vi "打码软件.vi"() -> ()   [LabVIEW 2014]
uses:
  <vilib>/Instr/_visa.llb/VISA Configure Serial Port (Instr).vi
  <vilib>/ptbypt/NI_PtbyPt.lvlib
panel:
  in  "监控":bool
  out "选项卡控件":enum32{"主选项卡", "监控"}(tab)
  in  "输入打标码后五位\n如：S0001":string
  in  "确定":bool
  out "当前打标码":string
  in  "手动打标":bool
  in  "停止":bool
  in  "退出":bool
  in  "PLC状态":bool
  out "串口通讯":bool
  out "PLC通讯":bool
  in  "返回":bool
  out "初始化回复":string
  out "打标模式回复":string
  out "初始条码":string
  out "打标V1写入回复":string
  out "打标V3写入回复":string
  out "开始打标写入回复":string
  out "停止打标回复":string
  in  "自动打标":bool
  out "错误输出 2":errorcluster caption="错误输出"
  out "元素":u32
  out "初始化文件回复":string
  # "SIC 打 标 软 件"
  # "自定义条码"
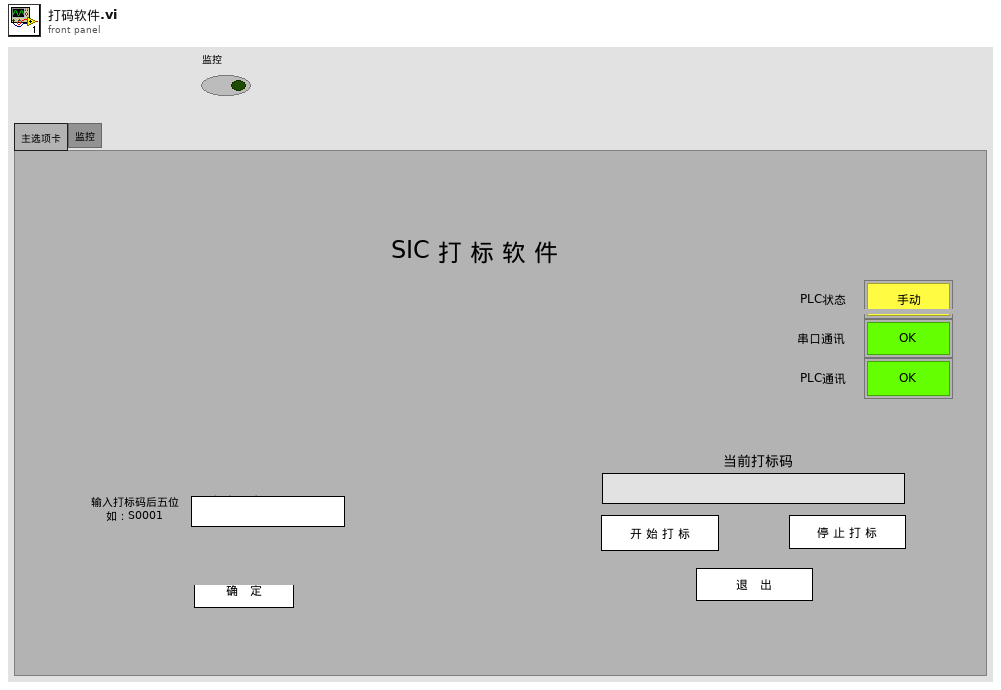
[diagram p1: front panel]
types:
  T1 = typedef "控件 1.ctl" = enum16{"通讯连接", "读PLC指令", "串口连接", "初始化", "打标模式", "事件", "错误", "退出"}
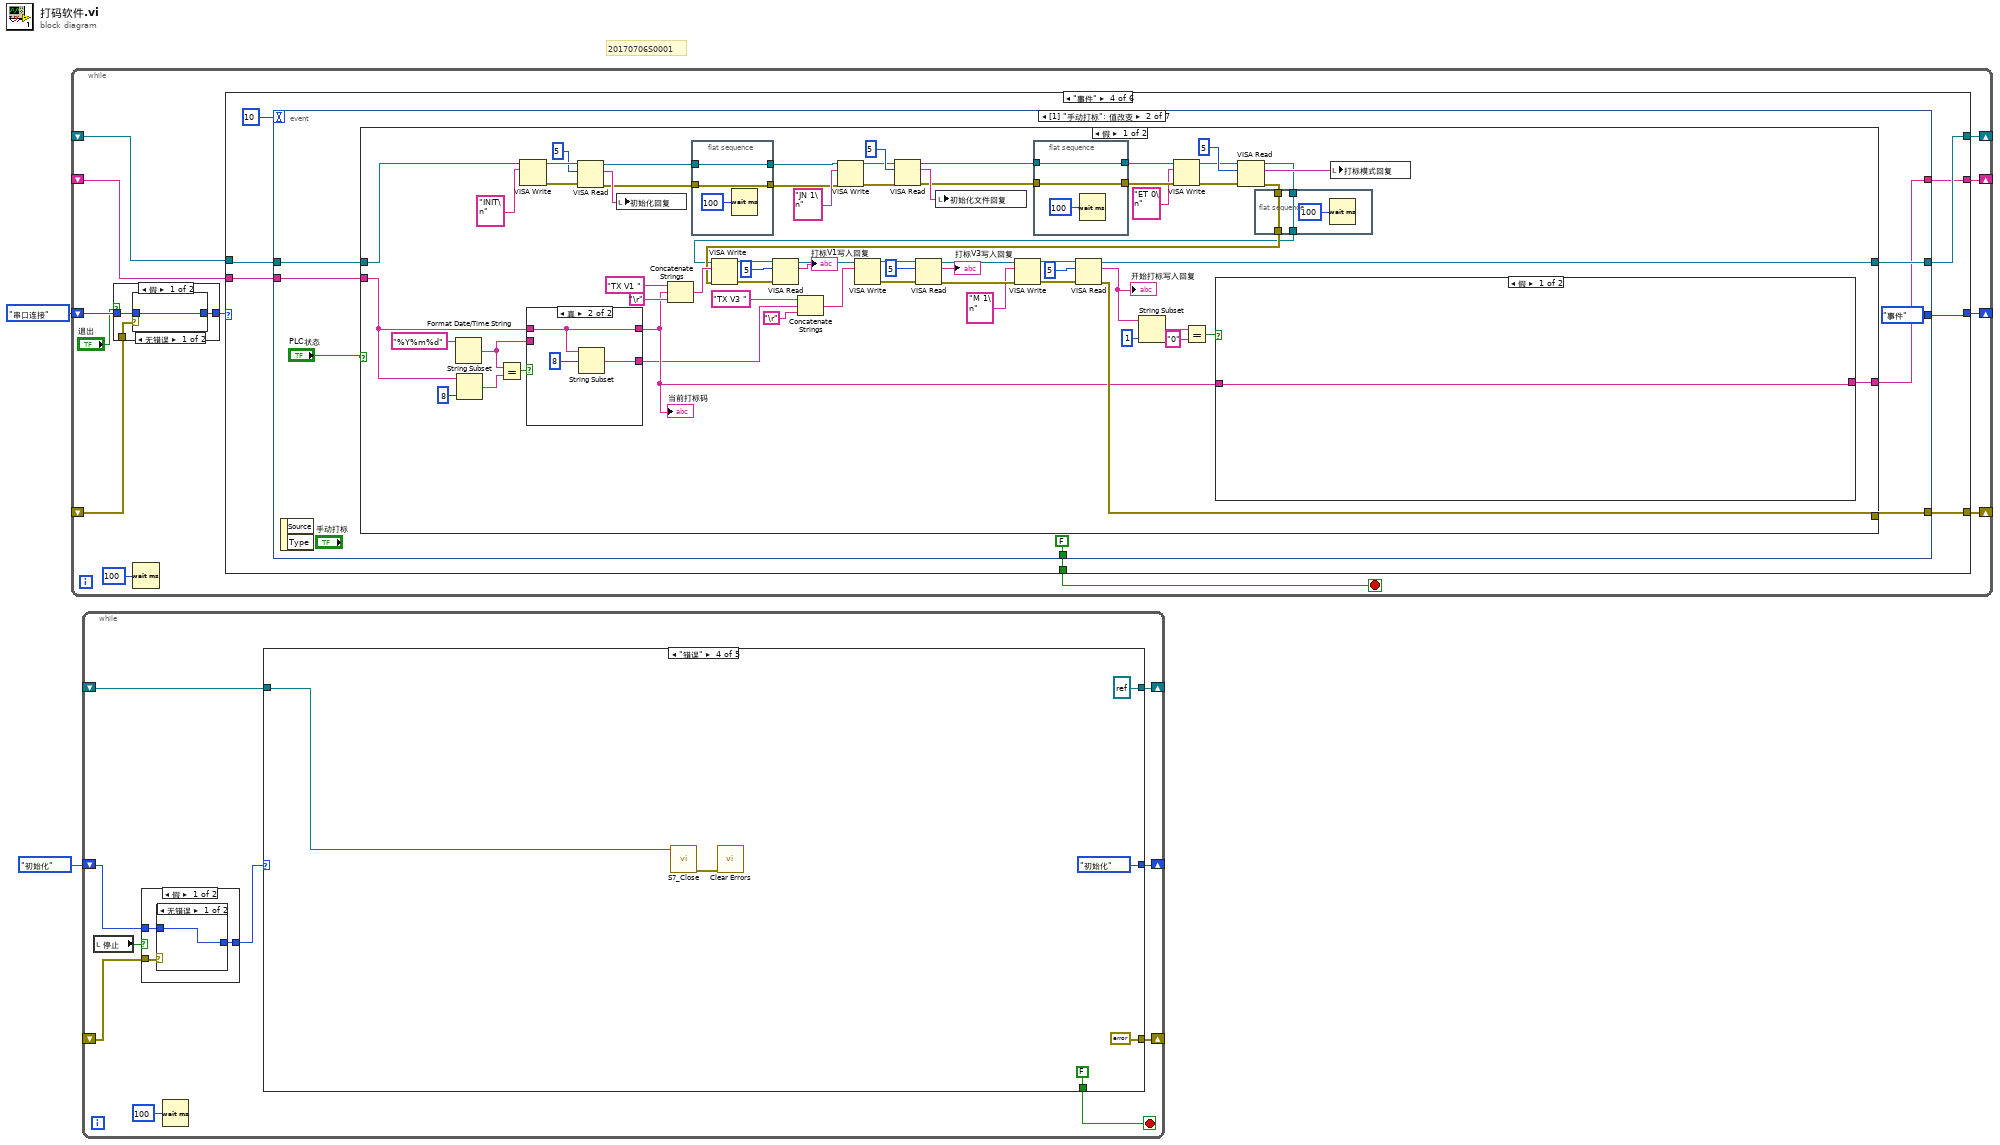
[diagram p0: block diagram]
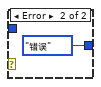
[diagram p2: hidden frame]
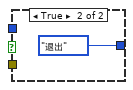
[diagram p3: hidden frame]
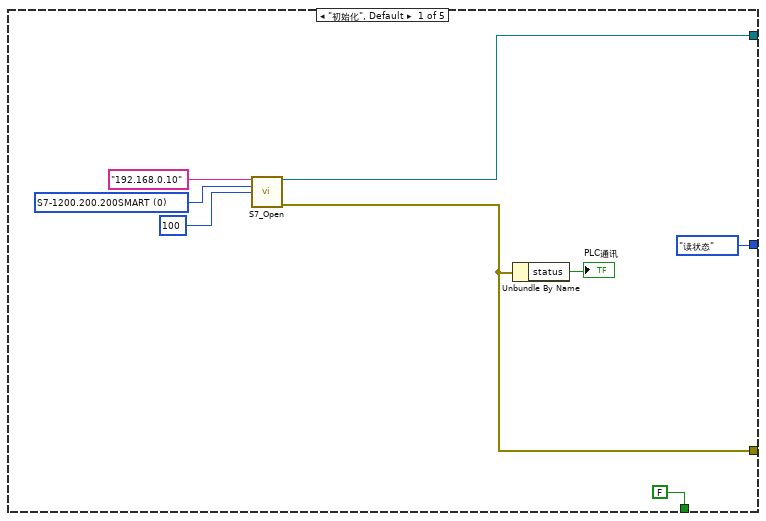
[diagram p4: hidden frame]
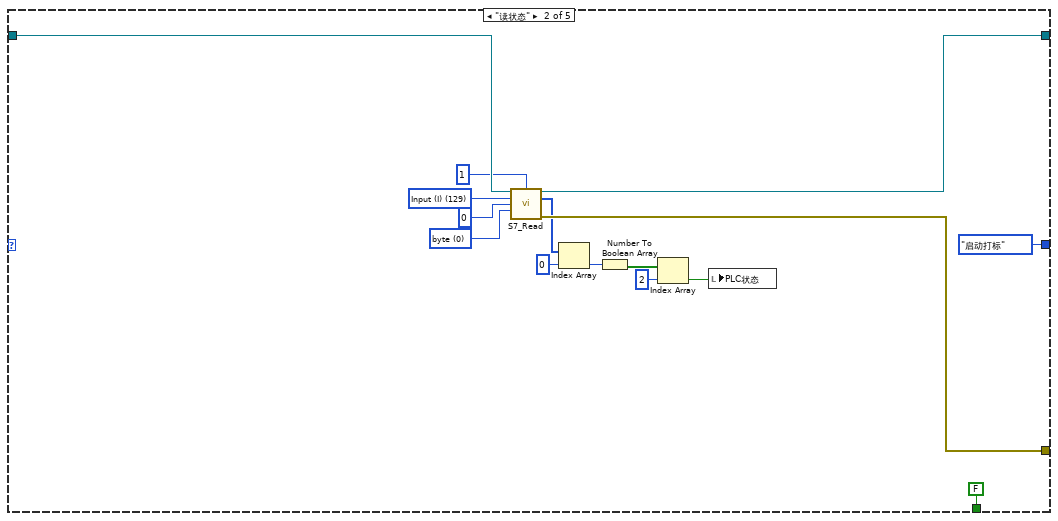
[diagram p5: hidden frame]
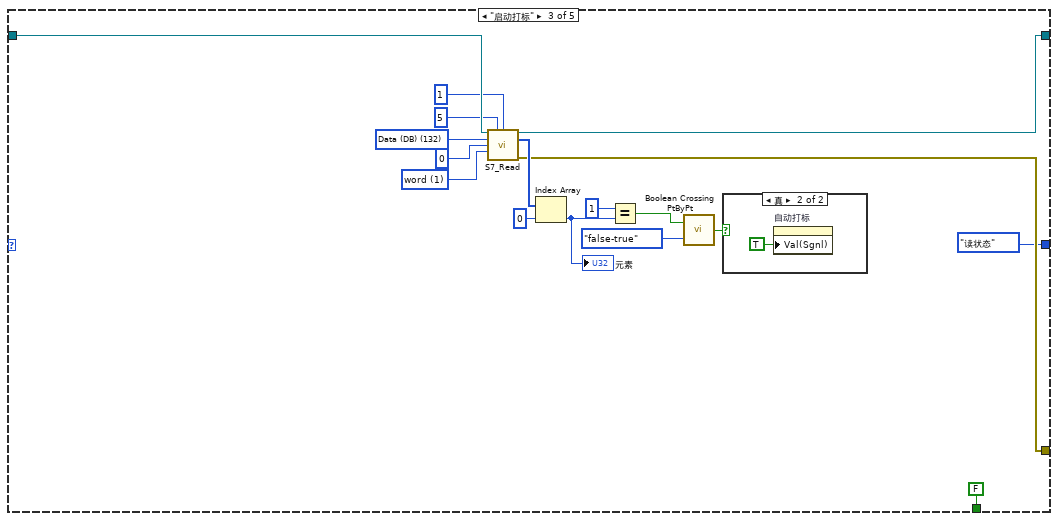
[diagram p6: hidden frame]
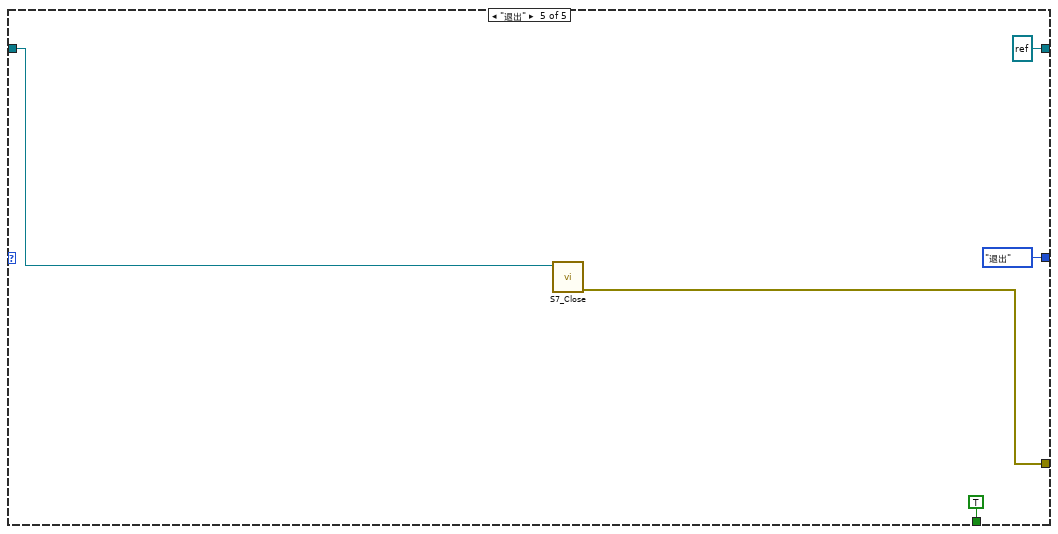
[diagram p8: hidden frame]
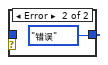
[diagram p9: hidden frame]
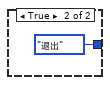
[diagram p10: hidden frame]
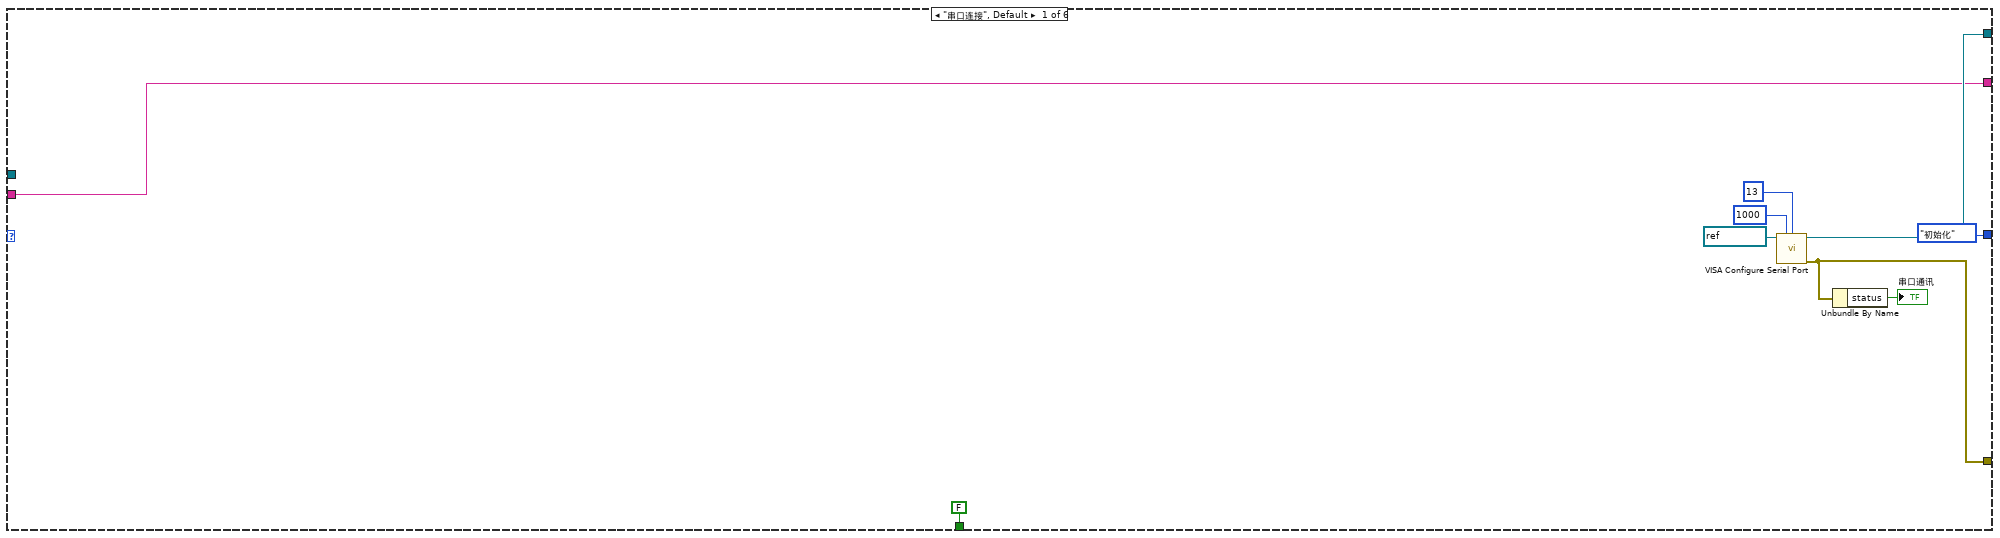
[diagram p11: hidden frame]
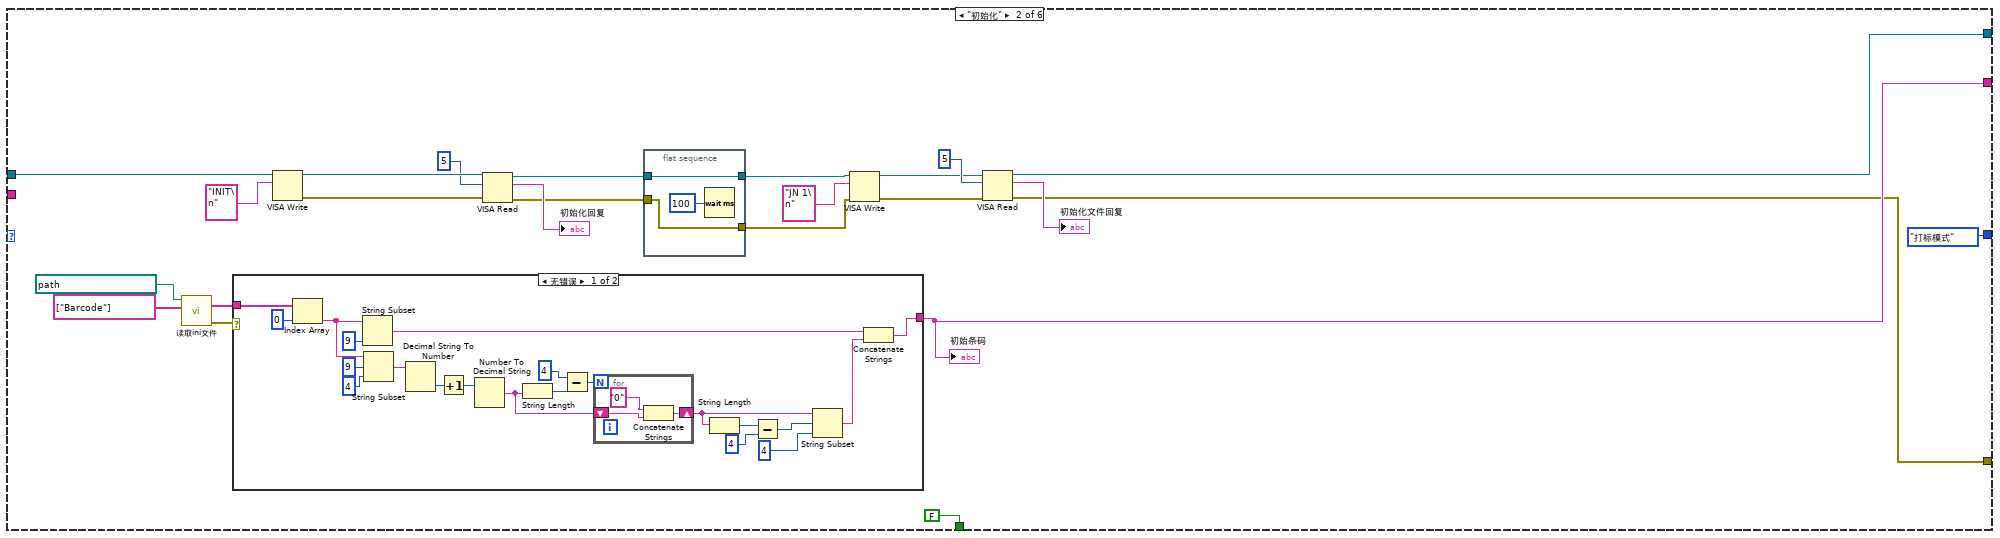
[diagram p12: hidden frame]
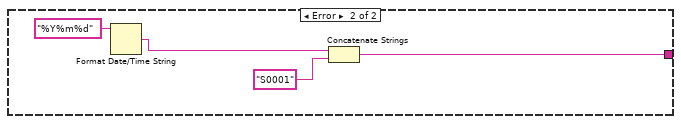
[diagram p13: hidden frame]
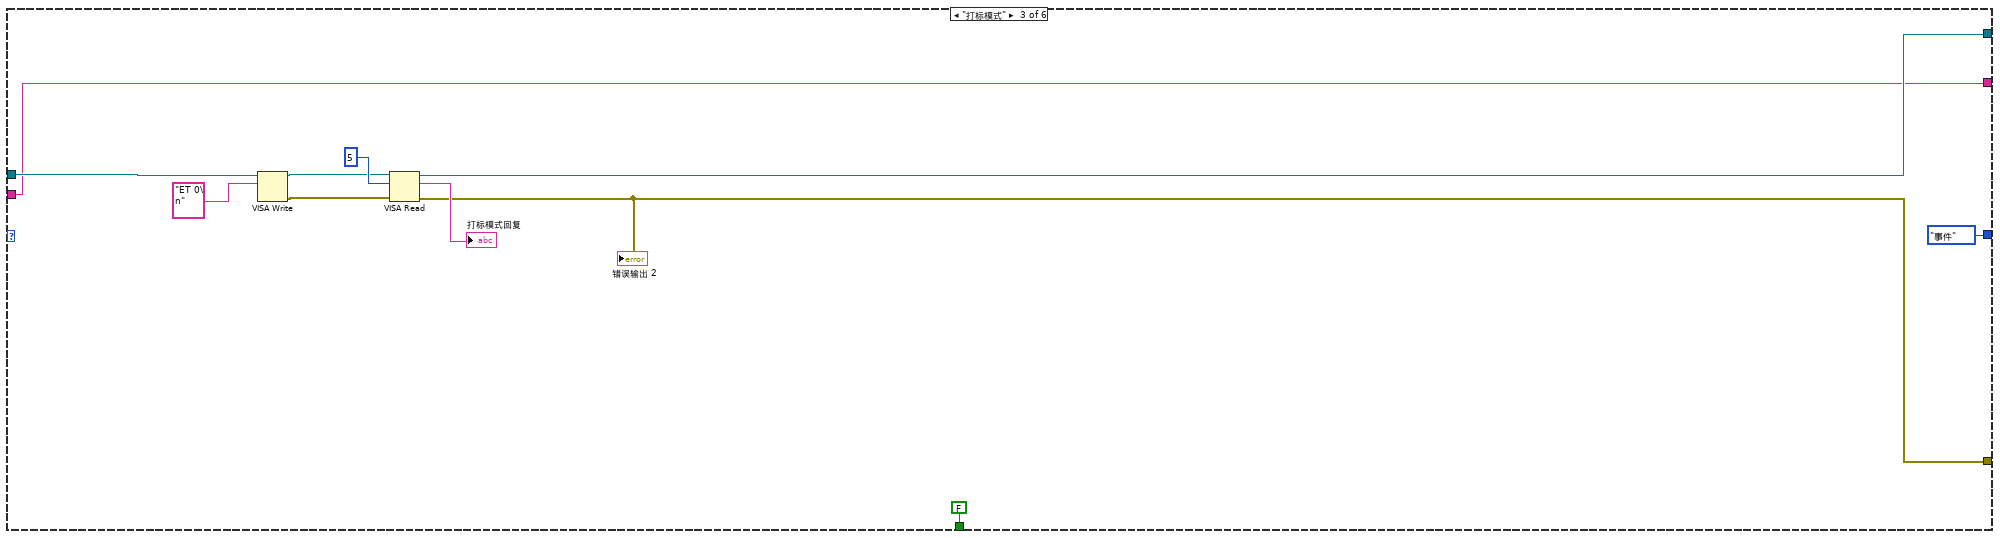
[diagram p14: hidden frame]
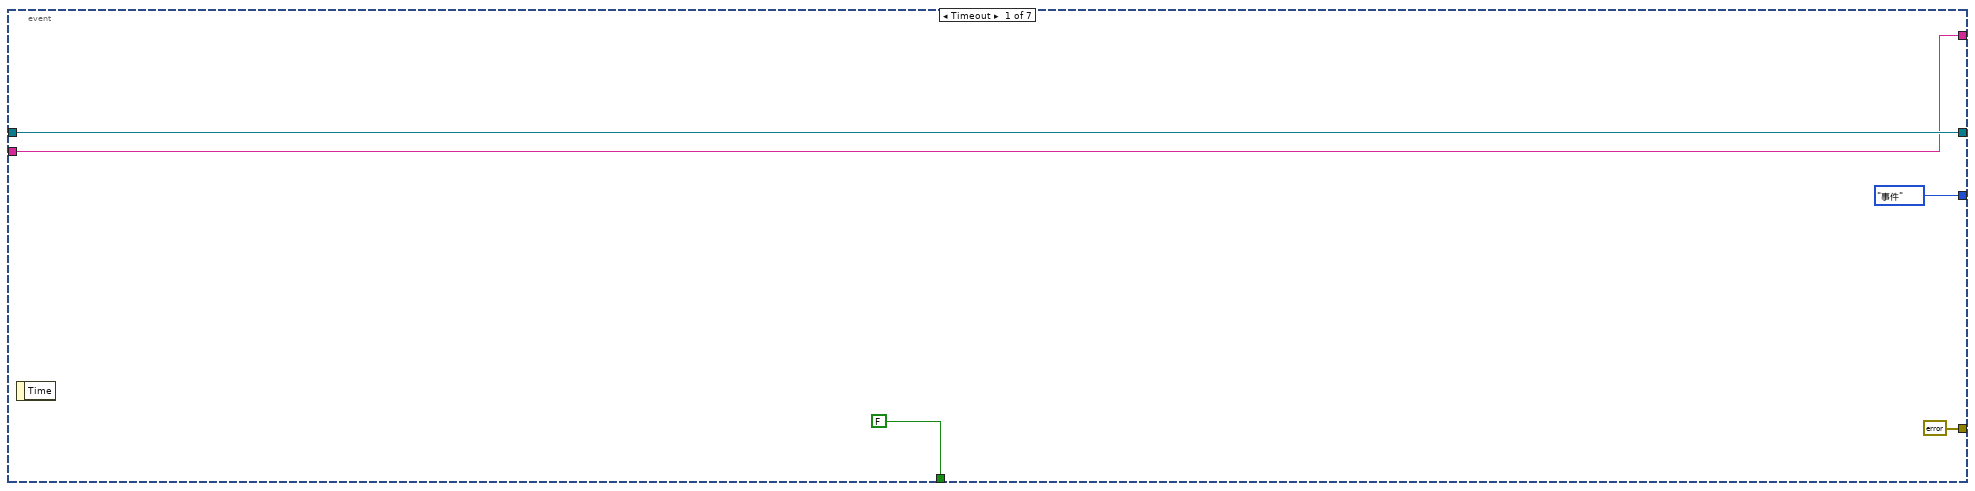
[diagram p15: hidden frame]
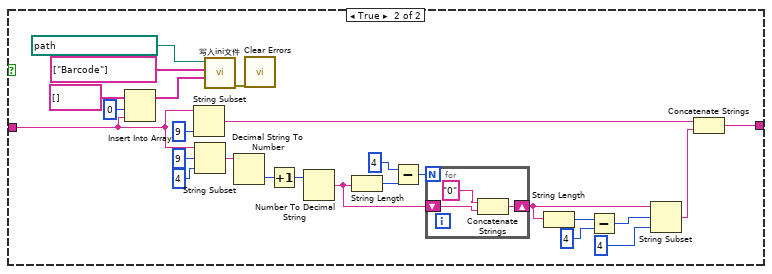
[diagram p16: hidden frame]
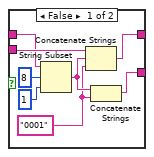
[diagram p17: hidden frame]
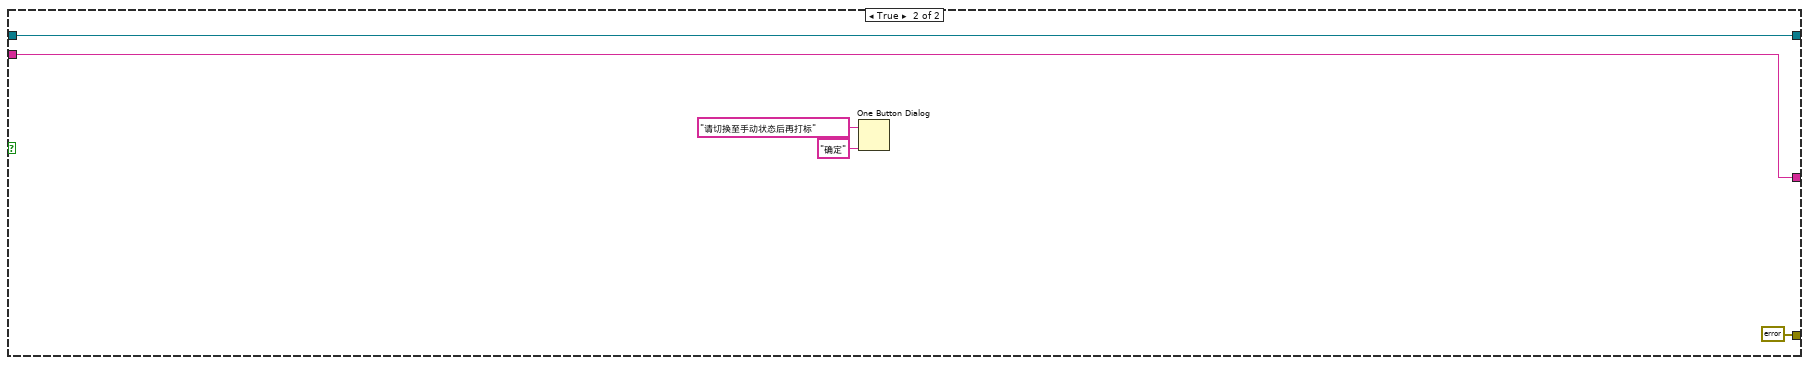
[diagram p18: hidden frame]
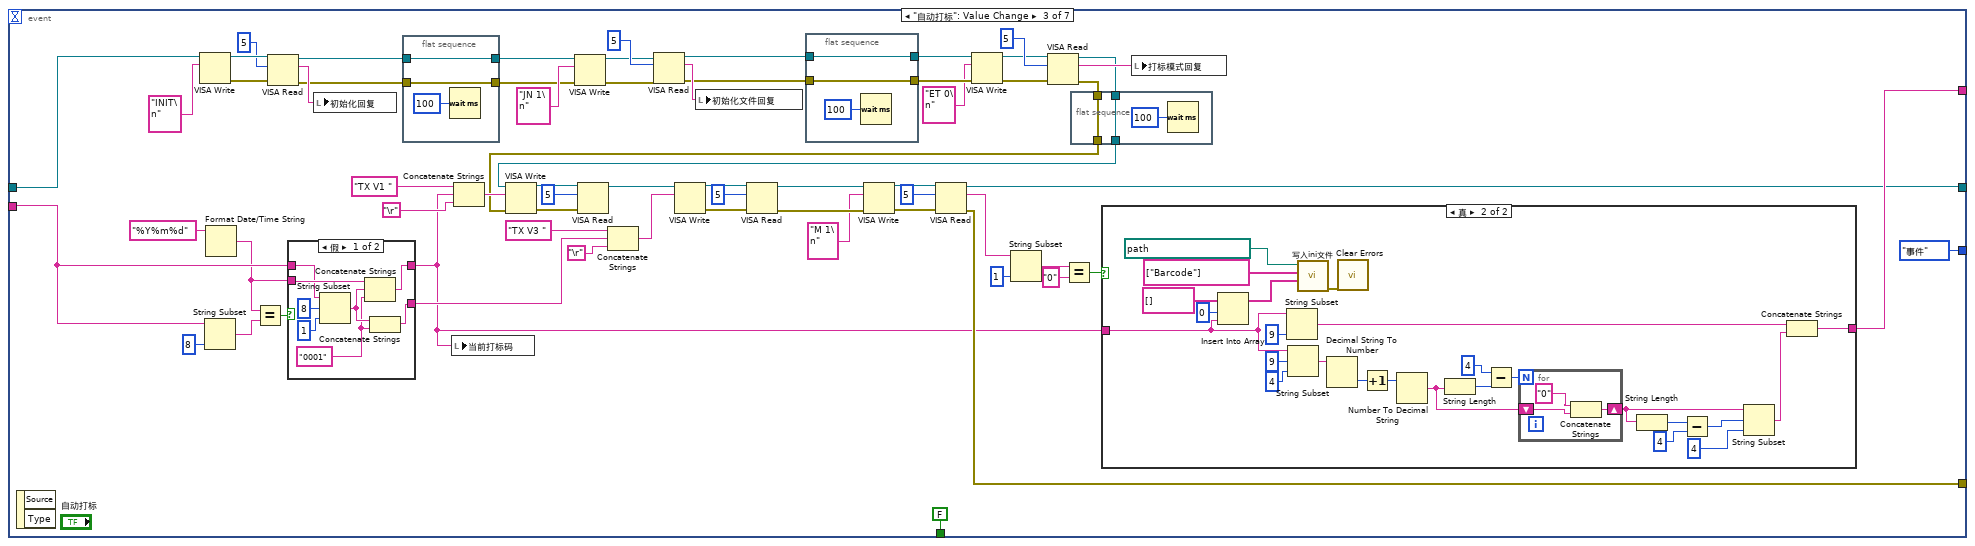
[diagram p19: hidden frame]
diagram:
  # "20170706S0001"
  n1 = while {
    shift-right: [w9] -> _
    shift-left: 控件_1."串口连接" -> [w14]
    shift-right: [w10] -> _
    shift-left: _ -> [w13]
    shift-right: [w11] -> _
    shift-left: _ -> [w8]
    shift-right: [w7] -> _
    shift-left: _ -> [w5]
    stop <- w6 stop-if-true
    n2 = case shown="假" "退出" {
      tunnel: w14 -> [w17 _]
      tunnel: w13 -> [w16 _]
      tunnel: [w15 控件_1."退出"] -> w12
      frame False {
        n3 = case shown="无错误" w16 {
          tunnel: w17 -> [w18 _]
          tunnel: [w18 控件_1."错误"] -> w15
          frame No Error {
          }
          frame Error {
          }
        }
      }
      frame True {
      }
    }
    n4 = Wait (ms)(milliseconds to wait=u32 100 ("等待时间（毫秒）")) -> ()  [unwired: 1 out]
    n5 = case shown="\"事件\"" w12 {
      tunnel: [w27 w31 w87 w99 refnum<visa-resource-name> refnum ("VISA resource name out") refnum<visa-resource-name> refnum ("VISA resource name out")] -> w11
      tunnel: [w24 w30 w88 w100 errorcluster {"status"=FALSE, "code"=0, "source"=""} ("error out") errorcluster {"status"=FALSE, "code"=0, "source"=""} ("error out")] -> w10
      tunnel: [控件_1."初始化" 控件_1."打标模式" 控件_1."事件" w97 控件_1."通讯连接" 控件_1."退出"] -> w9
      tunnel: w8 -> [_ w53 w94 w102 w386 w392]
      tunnel: [w22 w42 w85 w98 w384 ""] -> w7
      tunnel: [FALSE FALSE FALSE w96 FALSE TRUE] -> w6
      tunnel: w5 -> [w22 _ w85 w101 w384 _]
      frame "串口连接", Default {
        n6 = call-poly "VISA Configure Serial Port"("VISA resource name"=refnum<visa-resource-name> "COM1", "timeout (10sec)"=u32 1000, "termination char\n(0xA = '\\n' = LF)"=u8 13 ("termination char\n(0xA = '\\n' = LF)")) -> ("VISA resource name out"=w27:refnum<visa-resource-name>, "error out"=w24:errorcluster)  [unwired: 11 in]
        n7 = Unbundle By Name(w24) -> ("status"=→"串口通讯":bool)
      }
      frame "初始化" {
        n8 = call "读取ini文件.vi"("名称"=string[] ["Barcode"], "configuration file path"=path "D:/初始化文件/10.ini") -> ("error out"=w43:errorcluster, "值"=w44:string[])  [unwired: 8 in]
        n9 = case shown="无错误" w43 {
          tunnel: w44 -> [w77 _]
          tunnel: [w57 w82] -> w42
          frame No Error {
            n10 = Index Array(array=w77, index=0 ("索引")) -> (element=w58:string)
            n11 = String Subset(string=w58, length (rest)=9 ("长度（剩余）")) -> (substring=w60:string)  [unwired: 1 in]
            n12 = String Subset(string=w58, offset (0)=9 ("偏移量(0)"), length (rest)=4 ("长度（剩余）")) -> (substring=w63:string)
            n13 = Decimal String To Number(string=w63) -> (number=w62:i32)  [unwired: 2 in, 1 out]
            n14 = Increment(x=w62) -> (x+1=w61:i32)
            n15 = Number To Decimal String(number=w61) -> (decimal integer string=w67:string)  [unwired: 1 in]
            n16 = String Length(string=w67) -> (length=w64:i32)
            n17 = Subtract(x=4, y=w64) -> (x-y=w66:i32)
            n18 = for {
              N: w66 -> [_]
              shift-right: [w80] -> w69
              shift-left: w67 -> [w79]
              n19 = Concatenate Strings("0" ("字符串"), w79) -> (w80:string)
            }
            n20 = String Length(string=w69) -> (length=w70:i32)
            n21 = Subtract(x=w70, y=4 ("x")) -> (x-y=w72:i32)
            n22 = String Subset(string=w69, offset (0)=w72, length (rest)=4 ("长度（剩余）")) -> (substring=w59:string)
            n23 = Concatenate Strings(w60, w59) -> (w57:string)
          }
          frame Error {
            n24 = Format Date/Time String(time format string (%c)="%Y%m%d" ("时间格式字符串(%c)")) -> (date/time string=w81:string)  [unwired: 2 in]
            n25 = Concatenate Strings(w81, "S0001" ("字符串")) -> (w82:string)
          }
        }
        "初始条码" <- w42
        n26 = VISA Write(VISA resource name=w53, write buffer="INIT\n" ("写入缓冲区")) -> (VISA resource name out=w50:refnum<visa-resource-name>, error out=w49:errorcluster)  [unwired: 1 in, 1 out]
        n27 = VISA Read(VISA resource name=w50, byte count=u32 5 ("字节总数"), error in (no error)=w49) -> (VISA resource name out=w37:refnum<visa-resource-name>, read buffer=→"初始化回复":string, error out=w35:errorcluster)  [unwired: 1 out]
        n28 = flat-sequence {
          tunnel: [w56] -> w36
          tunnel: w37 -> [w56]
          tunnel: w35 -> [w55]
          tunnel: [w55] -> w34
          frame #0 {
            n29 = Wait (ms)(milliseconds to wait=u32 100 ("等待时间（毫秒）")) -> ()  [unwired: 1 out]
          }
        }
        n30 = VISA Write(VISA resource name=w36, write buffer="JN 1\n" ("写入缓冲区"), error in (no error)=w34) -> (VISA resource name out=w33:refnum<visa-resource-name>, error out=w32:errorcluster)  [unwired: 1 out]
        n31 = VISA Read(VISA resource name=w33, byte count=u32 5 ("字节总数"), error in (no error)=w32) -> (VISA resource name out=w31:refnum<visa-resource-name>, read buffer=→"初始化文件回复":string, error out=w30:errorcluster)  [unwired: 1 out]
      }
      frame "打标模式" {
        n32 = VISA Write(VISA resource name=w94, write buffer="ET 0\n" ("写入缓冲区")) -> (VISA resource name out=w89:refnum<visa-resource-name>, error out=w90:errorcluster)  [unwired: 1 in, 1 out]
        n33 = VISA Read(VISA resource name=w89, byte count=u32 5 ("字节总数"), error in (no error)=w90) -> (VISA resource name out=w87:refnum<visa-resource-name>, read buffer=→"打标模式回复":string, error out=w88:errorcluster)  [unwired: 1 out]
        "错误输出 2" <- w88
      }
      frame "事件" {
        n34 = event shown="[1] \"手动打标\": 值改变" {
          selector: _ -> [_ _ _ _ _ _ _]
          dyn-events: _ -> [_ _ _ _ _ _ _]
          timeout: 10 -> [_ _ _ _ _ _ _]
          tunnel: w102 -> [w108 w116 w240 w356 w365 w373 w378]
          tunnel: w101 -> [w107 w115 w269 w352 _ w374 w377]
          tunnel: [errorcluster {"status"=FALSE, "code"=0, "source"=""} ("error out") w114 w268 w353 errorcluster {"status"=FALSE, "code"=0, "source"=""} ("error out") errorcluster {"status"=FALSE, "code"=0, "source"=""} ("error out") errorcluster {"status"=FALSE, "code"=0, "source"=""} ("error out")] -> w100
          tunnel: [w108 w113 w266 w354 w365 w373 w378] -> w99
          tunnel: [w107 w112 w267 w352 w366 w374 w377] -> w98
          tunnel: [控件_1."事件" 控件_1."事件" 控件_1."事件" 控件_1."事件" 控件_1."事件" 控件_1."事件" 控件_1."事件"] -> w97
          tunnel: [FALSE FALSE FALSE FALSE FALSE FALSE FALSE] -> w96
          event Timeout {
            n35 = event-data() -> ()  [unwired: 1 in, 1 out]
          }
          event "手动打标": Value Change {
            n36 = event-data() -> ()  [unwired: 1 in, 2 out]
            n37 = case shown="假" "PLC状态" {
              tunnel: w116 -> [w121 w234]
              tunnel: w115 -> [w173 w235]
              tunnel: [w150 errorcluster {"status"=FALSE, "code"=0, "source"=""} ("error out")] -> w114
              tunnel: [w149 w234] -> w113
              tunnel: [w147 w235] -> w112
              frame False {
                n38 = Format Date/Time String(time format string (%c)="%Y%m%d" ("时间格式字符串(%c)")) -> (date/time string=w146:string)  [unwired: 2 in]
                n39 = String Subset(string=w173, length (rest)=8 ("长度（剩余）")) -> (substring=w175:string)  [unwired: 1 in]
                n40 = Equal?(x=w146, y=w175) -> (x = y?=w174:bool)
                n41 = VISA Write(VISA resource name=w121, write buffer="INIT\n" ("写入缓冲区")) -> (VISA resource name out=w132:refnum<visa-resource-name>, error out=w131:errorcluster)  [unwired: 1 in, 1 out]
                n42 = case shown="真" w174 {
                  tunnel: w173 -> [w226 w230]
                  tunnel: [w223 w230] -> w148
                  tunnel: [w222 w228] -> w145
                  tunnel: w146 -> [w227 _]
                  frame False {
                    w220 = "0001"
                    n43 = String Subset(string=w226, offset (0)=8 ("偏移量(0)"), length (rest)=1 ("长度（剩余）")) -> (substring=w221:string)
                    n44 = Concatenate Strings(w227, w221, w220) -> (w223:string)
                    n45 = Concatenate Strings(w221, w220) -> (w222:string)
                  }
                  frame True {
                    n46 = String Subset(string=w230, offset (0)=8 ("偏移量(0)")) -> (substring=w228:string)  [unwired: 1 in]
                  }
                }
                "当前打标码" <- w148
                n47 = VISA Read(VISA resource name=w132, byte count=u32 5 ("字节总数"), error in (no error)=w131) -> (VISA resource name out=w127:refnum<visa-resource-name>, read buffer=w142:string, error out=w125:errorcluster)  [unwired: 1 out]
                n48 = local write "初始化回复"(w142) -> ()
                n49 = Concatenate Strings("TX V1 " ("写入缓冲区"), w148, "\r") -> (w170:string)
                n50 = flat-sequence {
                  tunnel: [w190] -> w126
                  tunnel: w127 -> [w190]
                  tunnel: w125 -> [w189]
                  tunnel: [w189] -> w124
                  frame #0 {
                    n51 = Wait (ms)(milliseconds to wait=u32 100 ("等待时间（毫秒）")) -> ()  [unwired: 1 out]
                  }
                }
                n52 = VISA Write(VISA resource name=w117, write buffer=w170, error in (no error)=w119) -> (VISA resource name out=w181:refnum<visa-resource-name>, error out=w180:errorcluster)  [unwired: 1 out]
                n53 = VISA Read(VISA resource name=w181, byte count=u32 5 ("字节总数"), error in (no error)=w180) -> (VISA resource name out=w163:refnum<visa-resource-name>, read buffer=→"打标V1写入回复":string)  [unwired: 2 out]
                n54 = Concatenate Strings("TX V3 " ("写入缓冲区"), w145, "\r") -> (w169:string)
                n55 = VISA Write(VISA resource name=w126, write buffer="JN 1\n" ("写入缓冲区"), error in (no error)=w124) -> (VISA resource name out=w123:refnum<visa-resource-name>, error out=w122:errorcluster)  [unwired: 1 out]
                n56 = VISA Write(VISA resource name=w163, write buffer=w169) -> (VISA resource name out=w164:refnum<visa-resource-name>, error out=w165:errorcluster)  [unwired: 1 in, 1 out]
                n57 = VISA Read(VISA resource name=w123, byte count=u32 5 ("字节总数"), error in (no error)=w122) -> (VISA resource name out=w138:refnum<visa-resource-name>, read buffer=w143:string, error out=w140:errorcluster)  [unwired: 1 out]
                n58 = VISA Read(VISA resource name=w164, byte count=u32 5 ("字节总数"), error in (no error)=w165) -> (VISA resource name out=w158:refnum<visa-resource-name>, read buffer=→"打标V3写入回复":string, error out=w157:errorcluster)  [unwired: 1 out]
                n59 = local write "初始化文件回复"(w143) -> ()
                n60 = VISA Write(VISA resource name=w158, write buffer="M 1\n" ("写入缓冲区"), error in (no error)=w157) -> (VISA resource name out=w161:refnum<visa-resource-name>, error out=w160:errorcluster)  [unwired: 1 out]
                n61 = flat-sequence {
                  tunnel: [w187] -> w139
                  tunnel: w138 -> [w187]
                  tunnel: [w186] -> w141
                  tunnel: w140 -> [w186]
                  frame #0 {
                    n62 = Wait (ms)(milliseconds to wait=u32 100 ("等待时间（毫秒）")) -> ()  [unwired: 1 out]
                  }
                }
                n63 = VISA Read(VISA resource name=w161, byte count=u32 5 ("字节总数"), error in (no error)=w160) -> (VISA resource name out=w149:refnum<visa-resource-name>, read buffer=w155:string, error out=w150:errorcluster)  [unwired: 1 out]
                "开始打标写入回复" <- w155
                n64 = String Subset(string=w155, length (rest)=1 ("长度（剩余）")) -> (substring=w153:string)  [unwired: 1 in]
                n65 = VISA Write(VISA resource name=w139, write buffer="ET 0\n" ("写入缓冲区"), error in (no error)=w141) -> (VISA resource name out=w134:refnum<visa-resource-name>, error out=w135:errorcluster)  [unwired: 1 out]
                n66 = Equal?(x=w153, y="0") -> (x = y?=w151:bool)
                n67 = case shown="假" w151 {
                  tunnel: w148 -> [w191 w193]
                  tunnel: [w191 w192] -> w147
                  frame False {
                  }
                  frame True {
                    n68 = Insert Into Array(array=string[] [] ("数组"), index=0 ("索引"), new element=w193) -> (w213:string[])
                    n69 = String Subset(string=w193, length (rest)=9 ("长度（剩余）")) -> (substring=w195:string)  [unwired: 1 in]
                    n70 = String Subset(string=w193, offset (0)=9 ("偏移量(0)"), length (rest)=4 ("长度（剩余）")) -> (substring=w198:string)
                    n71 = call "写入ini文件.vi"("值"=w213, "名称"=string[] ["Barcode"], "configuration file path"=path "D:/初始化文件/10.ini") -> ("error out"=w216:errorcluster)  [unwired: 8 in]
                    n72 = Decimal String To Number(string=w198) -> (number=w197:i32)  [unwired: 2 in, 1 out]
                    n73 = call <vilib>:"Clear Errors.vi"("error in (no error)"=w216) -> ()  [unwired: 5 in, 2 out]
                    n74 = Increment(x=w197) -> (x+1=w196:i32)
                    n75 = Number To Decimal String(number=w196) -> (decimal integer string=w202:string)  [unwired: 1 in]
                    n76 = String Length(string=w202) -> (length=w199:i32)
                    n77 = Subtract(x=4, y=w199) -> (x-y=w201:i32)
                    n78 = for {
                      N: w201 -> [_]
                      shift-right: [w219] -> w204
                      shift-left: w202 -> [w218]
                      n79 = Concatenate Strings("0" ("字符串"), w218) -> (w219:string)
                    }
                    n80 = String Length(string=w204) -> (length=w205:i32)
                    n81 = Subtract(x=w205, y=4 ("x")) -> (x-y=w207:i32)
                    n82 = String Subset(string=w204, offset (0)=w207, length (rest)=4 ("长度（剩余）")) -> (substring=w194:string)
                    n83 = Concatenate Strings(w195, w194) -> (w192:string)
                  }
                }
                n84 = VISA Read(VISA resource name=w134, byte count=u32 5 ("字节总数"), error in (no error)=w135) -> (VISA resource name out=w118:refnum<visa-resource-name>, read buffer=w144:string, error out=w120:errorcluster)  [unwired: 1 out]
                n85 = flat-sequence {
                  tunnel: w118 -> [w184]
                  tunnel: [w184] -> w117
                  tunnel: w120 -> [w183]
                  tunnel: [w183] -> w119
                  frame #0 {
                    n86 = Wait (ms)(milliseconds to wait=u32 100 ("等待时间（毫秒）")) -> ()  [unwired: 1 out]
                  }
                }
                n87 = local write "打标模式回复"(w144) -> ()
              }
              frame True {
                n88 = One Button Dialog(message="请切换至手动状态后再打标" ("消息"), button name ("OK")="确定" ("按钮名称（“确定”）")) -> ()  [unwired: 1 out]
              }
            }
          }
          event "自动打标": Value Change {
            n89 = event-data() -> ()  [unwired: 1 in, 2 out]
            n90 = VISA Write(VISA resource name=w240, write buffer="INIT\n" ("写入缓冲区")) -> (VISA resource name out=w251:refnum<visa-resource-name>, error out=w250:errorcluster)  [unwired: 1 in, 1 out]
            n91 = String Subset(string=w269, length (rest)=8 ("长度（剩余）")) -> (substring=w293:string)  [unwired: 1 in]
            n92 = Format Date/Time String(time format string (%c)="%Y%m%d" ("时间格式字符串(%c)")) -> (date/time string=w264:string)  [unwired: 2 in]
            n93 = Equal?(x=w264, y=w293) -> (x = y?=w292:bool)
            n94 = VISA Read(VISA resource name=w251, byte count=u32 5 ("字节总数"), error in (no error)=w250) -> (VISA resource name out=w246:refnum<visa-resource-name>, read buffer=w261:string, error out=w244:errorcluster)  [unwired: 1 out]
            n95 = case shown="假" w292 {
              tunnel: w269 -> [w345 w349]
              tunnel: [w342 w349] -> w265
              tunnel: [w341 w347] -> w281
              tunnel: w264 -> [w346 _]
              frame False {
                w339 = "0001"
                n96 = String Subset(string=w345, offset (0)=8 ("偏移量(0)"), length (rest)=1 ("长度（剩余）")) -> (substring=w340:string)
                n97 = Concatenate Strings(w346, w340, w339) -> (w342:string)
                n98 = Concatenate Strings(w340, w339) -> (w341:string)
              }
              frame True {
                n99 = String Subset(string=w349, offset (0)=8 ("偏移量(0)")) -> (substring=w347:string)  [unwired: 1 in]
              }
            }
            n100 = local write "初始化回复"(w261) -> ()
            n101 = flat-sequence {
              tunnel: [w309] -> w245
              tunnel: w246 -> [w309]
              tunnel: w244 -> [w308]
              tunnel: [w308] -> w243
              frame #0 {
                n102 = Wait (ms)(milliseconds to wait=u32 100 ("等待时间（毫秒）")) -> ()  [unwired: 1 out]
              }
            }
            n103 = local write "当前打标码"(w265) -> ()
            n104 = Concatenate Strings("TX V1 " ("写入缓冲区"), w265, "\r") -> (w289:string)
            n105 = VISA Write(VISA resource name=w238, write buffer=w289, error in (no error)=w236) -> (VISA resource name out=w298:refnum<visa-resource-name>, error out=w297:errorcluster)  [unwired: 1 out]
            n106 = VISA Write(VISA resource name=w245, write buffer="JN 1\n" ("写入缓冲区"), error in (no error)=w243) -> (VISA resource name out=w242:refnum<visa-resource-name>, error out=w241:errorcluster)  [unwired: 1 out]
            n107 = VISA Read(VISA resource name=w298, byte count=u32 5 ("字节总数"), error in (no error)=w297) -> (VISA resource name out=w282:refnum<visa-resource-name>)  [unwired: 3 out]
            n108 = Concatenate Strings("TX V3 " ("写入缓冲区"), w281, "\r") -> (w288:string)
            n109 = VISA Read(VISA resource name=w242, byte count=u32 5 ("字节总数"), error in (no error)=w241) -> (VISA resource name out=w257:refnum<visa-resource-name>, read buffer=w262:string, error out=w259:errorcluster)  [unwired: 1 out]
            n110 = VISA Write(VISA resource name=w282, write buffer=w288) -> (VISA resource name out=w283:refnum<visa-resource-name>, error out=w284:errorcluster)  [unwired: 1 in, 1 out]
            n111 = local write "初始化文件回复"(w262) -> ()
            n112 = VISA Read(VISA resource name=w283, byte count=u32 5 ("字节总数"), error in (no error)=w284) -> (VISA resource name out=w277:refnum<visa-resource-name>, error out=w276:errorcluster)  [unwired: 2 out]
            n113 = flat-sequence {
              tunnel: [w306] -> w258
              tunnel: w257 -> [w306]
              tunnel: [w305] -> w260
              tunnel: w259 -> [w305]
              frame #0 {
                n114 = Wait (ms)(milliseconds to wait=u32 100 ("等待时间（毫秒）")) -> ()  [unwired: 1 out]
              }
            }
            n115 = VISA Write(VISA resource name=w277, write buffer="M 1\n" ("写入缓冲区"), error in (no error)=w276) -> (VISA resource name out=w280:refnum<visa-resource-name>, error out=w279:errorcluster)  [unwired: 1 out]
            n116 = VISA Read(VISA resource name=w280, byte count=u32 5 ("字节总数"), error in (no error)=w279) -> (VISA resource name out=w266:refnum<visa-resource-name>, read buffer=w274:string, error out=w268:errorcluster)  [unwired: 1 out]
            n117 = VISA Write(VISA resource name=w258, write buffer="ET 0\n" ("写入缓冲区"), error in (no error)=w260) -> (VISA resource name out=w253:refnum<visa-resource-name>, error out=w254:errorcluster)  [unwired: 1 out]
            n118 = String Subset(string=w274, length (rest)=1 ("长度（剩余）")) -> (substring=w272:string)  [unwired: 1 in]
            n119 = VISA Read(VISA resource name=w253, byte count=u32 5 ("字节总数"), error in (no error)=w254) -> (VISA resource name out=w239:refnum<visa-resource-name>, read buffer=w263:string, error out=w237:errorcluster)  [unwired: 1 out]
            n120 = Equal?(x=w272, y="0") -> (x = y?=w270:bool)
            n121 = flat-sequence {
              tunnel: w239 -> [w303]
              tunnel: [w303] -> w238
              tunnel: w237 -> [w302]
              tunnel: [w302] -> w236
              frame #0 {
                n122 = Wait (ms)(milliseconds to wait=u32 100 ("等待时间（毫秒）")) -> ()  [unwired: 1 out]
              }
            }
            n123 = case shown="真" w270 {
              tunnel: w265 -> [w310 w312]
              tunnel: [w310 w311] -> w267
              frame False {
              }
              frame True {
                n124 = Insert Into Array(array=string[] [] ("数组"), index=0 ("索引"), new element=w312) -> (w332:string[])
                n125 = String Subset(string=w312, length (rest)=9 ("长度（剩余）")) -> (substring=w314:string)  [unwired: 1 in]
                n126 = String Subset(string=w312, offset (0)=9 ("偏移量(0)"), length (rest)=4 ("长度（剩余）")) -> (substring=w317:string)
                n127 = call "写入ini文件.vi"("值"=w332, "名称"=string[] ["Barcode"], "configuration file path"=path "D:/初始化文件/10.ini") -> ("error out"=w335:errorcluster)  [unwired: 8 in]
                n128 = Decimal String To Number(string=w317) -> (number=w316:i32)  [unwired: 2 in, 1 out]
                n129 = call <vilib>:"Clear Errors.vi"("error in (no error)"=w335) -> ()  [unwired: 5 in, 2 out]
                n130 = Increment(x=w316) -> (x+1=w315:i32)
                n131 = Number To Decimal String(number=w315) -> (decimal integer string=w321:string)  [unwired: 1 in]
                n132 = String Length(string=w321) -> (length=w318:i32)
                n133 = Subtract(x=4, y=w318) -> (x-y=w320:i32)
                n134 = for {
                  N: w320 -> [_]
                  shift-right: [w338] -> w323
                  shift-left: w321 -> [w337]
                  n135 = Concatenate Strings("0" ("字符串"), w337) -> (w338:string)
                }
                n136 = String Length(string=w323) -> (length=w324:i32)
                n137 = Subtract(x=w324, y=4 ("x")) -> (x-y=w326:i32)
                n138 = String Subset(string=w323, offset (0)=w326, length (rest)=4 ("长度（剩余）")) -> (substring=w313:string)
                n139 = Concatenate Strings(w314, w313) -> (w311:string)
              }
            }
            n140 = local write "打标模式回复"(w263) -> ()
          }
          event "停止": Value Change {
            n141 = event-data() -> ()  [unwired: 1 in, 2 out]
            n142 = VISA Write(VISA resource name=w356, write buffer="M 0\n" ("写入缓冲区")) -> (VISA resource name out=w360:refnum<visa-resource-name>, error out=w359:errorcluster)  [unwired: 1 in, 1 out]
            n143 = VISA Read(VISA resource name=w360, byte count=u32 5 ("字节总数"), error in (no error)=w359) -> (VISA resource name out=w354:refnum<visa-resource-name>, read buffer=→"停止打标回复":string, error out=w353:errorcluster)  [unwired: 1 out]
          }
          event "确定": Value Change {
            n144 = event-data() -> ()  [unwired: 1 in, 2 out]
            n145 = Format Date/Time String(time format string (%c)="%Y%m%d" ("时间格式字符串(%c)")) -> (date/time string=w361:string)  [unwired: 2 in]
            n146 = Concatenate Strings(w361, "输入打标码后五位\n如：S0001") -> (w366:string)
          }
          event "监控": Value Change {
            n147 = event-data() -> ()  [unwired: 1 in, 4 out]
            "选项卡控件" <- enum32{"主选项卡", "监控"}."监控" ("选项卡控件")
          }
          event "返回": Value Change {
            n148 = event-data() -> ()  [unwired: 1 in, 4 out]
            n149 = local write "选项卡控件"(enum32{"主选项卡", "监控"}."主选项卡" ("选项卡控件")) -> ()
          }
        }
      }
      frame "错误" {
        n150 = VISA Close(VISA resource name=w386) -> ()  [unwired: 1 in, 1 out]
      }
      frame "退出" {
        n151 = VISA Close(VISA resource name=w392) -> (error out=w393:errorcluster)  [unwired: 1 in]
        n152 = call <vilib>:"Clear Errors.vi"("error in (no error)"=w393) -> ()  [unwired: 5 in, 2 out]
        n153 = control-ref of="本VI"() -> (w394:refnum<vi>)
        n154 = invoke class="VI" method="FP.Close"(reference=w394) -> ()  [unwired: 2 in, 3 out]
      }
    }
  }
  n155 = while {
    shift-right: [w403] -> _
    shift-left: _ -> [w400]
    shift-right: [w402] -> _
    shift-left: _ -> [w398]
    shift-right: [w401] -> _
    shift-left: enum16{"初始化", "读状态", "启动打标", "错误", "退出"}."初始化" -> [w397]
    stop <- w399 stop-if-true
    n156 = local read "停止"() -> (w404:bool)
    n157 = case shown="假" w404 {
      tunnel: [w406 enum16{"初始化", "读状态", "启动打标", "错误", "退出"}."退出"] -> w396
      tunnel: w398 -> [w407 _]
      tunnel: w397 -> [w405 _]
      frame False {
        n158 = case shown="无错误" w407 {
          tunnel: [w408 enum16{"初始化", "读状态", "启动打标", "错误", "退出"}."错误"] -> w406
          tunnel: w405 -> [w408 _]
          frame No Error {
          }
          frame Error {
          }
        }
      }
      frame True {
      }
    }
    n159 = Wait (ms)(milliseconds to wait=u32 100 ("等待时间（毫秒）")) -> ()  [unwired: 1 out]
    n160 = case shown="\"错误\"" w396 {
      tunnel: [w414 w428 w444 refnum<k5> refnum ("TCP") refnum<k5> refnum ("TCP")] -> w403
      tunnel: [w413 w429 w443 errorcluster {"status"=FALSE, "code"=0, "source"=""} ("error out") w461] -> w402
      tunnel: [enum16{"初始化", "读状态", "启动打标", "错误", "退出"}."读状态" enum16{"初始化", "读状态", "启动打标", "错误", "退出"}."启动打标" enum16{"初始化", "读状态", "启动打标", "错误", "退出"}."读状态" enum16{"初始化", "读状态", "启动打标", "错误", "退出"}."初始化" enum16{"初始化", "读状态", "启动打标", "错误", "退出"}."退出"] -> w401
      tunnel: w400 -> [_ w433 w445 w457 w462]
      tunnel: [FALSE FALSE FALSE FALSE TRUE] -> w399
      frame "初始化", Default {
        w417 = u8 0 items=["S7-1200.200.200SMART"=0, "S7-300"=2, "S7-400"=3] ("PLC 系列")
        n161 = call "S7_Open.vi"("IP 地址"="192.168.0.10", "PLC 系列"=w417, "超时（MS）"=100) -> ("TCP"=w414:refnum<k5>, "error out"=w413:errorcluster)  [unwired: 10 in, 1 out]
        n162 = Unbundle By Name(w413) -> ("status"=→"PLC通讯":bool)
      }
      frame "读状态" {
        w430 = u16 0 items=["byte", "word", "Dword"] ("数据类型")
        w432 = u8 129 items=["I/O (P)"=128, "Input (I)"=129, "Output (Q)"=130, "Bit Memory (M)"=131, "Data (DB)"=132, "Instance Data (DI)"=133, "Local Data (L)"=134, "Predecessor Local Data (VL)"=135] ("寄存器类型")
        n163 = call "S7_Read.vi"("TCP"=w433, "读取长度"=u16 1, "寄存器类型"=w432, "起始地址"=u32 0, "数据类型"=w430) -> ("TCP"=w428:refnum<k5>, "数据"=w427:u32[], "error out"=w429:errorcluster)  [unwired: 7 in, 1 out]
        n164 = Index Array(array=w427, index=0 ("索引")) -> (element=w422:u32)
        n165 = Number To Boolean Array(number=w422) -> (Boolean array=w421:bool[])
        n166 = Index Array(array=w421, index=2 ("索引")) -> (element=w419:bool)
        n167 = local write "PLC状态"(w419) -> ()
      }
      frame "启动打标" {
        w448 = u16 1 items=["byte", "word", "Dword"] ("数据类型")
        w450 = u8 132 items=["I/O (P)"=128, "Input (I)"=129, "Output (Q)"=130, "Bit Memory (M)"=131, "Data (DB)"=132, "Instance Data (DI)"=133, "Local Data (L)"=134, "Predecessor Local Data (VL)"=135] ("寄存器类型")
        n168 = call "S7_Read.vi"("TCP"=w445, "DB #"=u16 5, "读取长度"=u16 1, "寄存器类型"=w450, "起始地址"=u32 0, "数据类型"=w448) -> ("TCP"=w444:refnum<k5>, "数据"=w447:u32[], "error out"=w443:errorcluster)  [unwired: 6 in, 1 out]
        n169 = Index Array(array=w447, index=0 ("索引")) -> (element=w436:u32)
        "元素" <- w436
        n170 = Equal?(x=u32 1, y=w436) -> (x = y?=w434:bool)
        n171 = call <vilib>:"Boolean Crossing PtByPt.vi"("direction"=enum16{"either", "false-true", "true-false"}."false-true", "input"=w434) -> ("crossing"=w439:bool)  [unwired: 1 in]
        n172 = case shown="真" w439 {
          frame False {
          }
          frame True {
            n173 = property on="自动打标" class="Bool (严格)"("Val(Sgnl)"=TRUE ("值(信号)")) -> ()  [unwired: 2 in, 2 out]
          }
        }
      }
      frame "错误" {
        n174 = call "S7_Close.vi"("TCP Connection Ref"=w457) -> ("error out"=w453:errorcluster)  [unwired: 10 in]
        n175 = call <vilib>:"Clear Errors.vi"("error in (no error)"=w453) -> ()  [unwired: 5 in, 2 out]
      }
      frame "退出" {
        n176 = call "S7_Close.vi"("TCP Connection Ref"=w462) -> ("error out"=w461:errorcluster)  [unwired: 10 in]
      }
    }
  }
